vi "Noyito10ChannelADC_CloseSerialPortConnection.vi"(8 "error in (no error)":errorcluster, 11 "Noyito 10Chan ADC Mod":refnum<visa-resource-name>) -> (0 "error out":errorcluster, 3 "Port Closed?":bool)   [LabVIEW 2020, in "NOYITO 10 Channel ADC Module Driver.lvlib"]
uses:
  NOYITO 10 Channel ADC Module Driver.lvlib
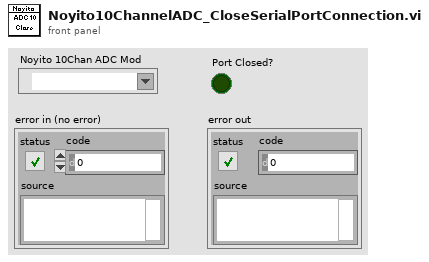
[diagram p1: front panel]
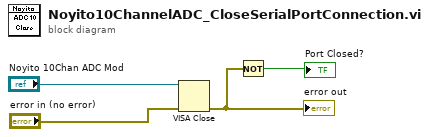
[diagram p0: block diagram]
diagram:
  n1 = VISA Close(VISA resource name="Noyito 10Chan ADC Mod", error in (no error)="error in (no error)") -> (error out=w2:errorcluster)
  "error out" <- w2
  n2 = Not(x=w2) -> (.not. x?=→"Port Closed?":bool)
